vi "Coloring B-Scan Demo.vi"() -> ()   [LabVIEW 2012]
uses:
  LabVIEW/user.lib/SpectralRadar.llb/Color Enhancement Selection.ctl
  LabVIEW/user.lib/SpectralRadar.llb/Colorscheme Selection.ctl
  LabVIEW/user.lib/SpectralRadar.llb/Coloring Byteorder.ctl
  LabVIEW/user.lib/SpectralRadar.llb/Device Camera Preset Selection.ctl
  LabVIEW/user.lib/SpectralRadar.llb/Processing Parameter Int Selection.ctl
  LabVIEW/user.lib/SpectralRadar.llb/Probe Parameter Int Selection.ctl
  LabVIEW/user.lib/SpectralRadar.llb/Colored Data Export Format Selection.ctl
  LabVIEW/user.lib/SpectralRadar.llb/set Transposed Colored Scan Output.vi
  LabVIEW/user.lib/SpectralRadar.llb/set Scan Output.vi
  LabVIEW/user.lib/SpectralRadar.llb/Data.lvclass
  LabVIEW/user.lib/SpectralRadar.llb/OCT Device.lvclass
  LabVIEW/user.lib/SpectralRadar.llb/Probe.lvclass
  LabVIEW/user.lib/SpectralRadar.llb/Processing.lvclass
  LabVIEW/user.lib/SpectralRadar.llb/Raw Data.lvclass
  LabVIEW/user.lib/SpectralRadar.llb/Scan Pattern.lvclass
  LabVIEW/user.lib/SpectralRadar.llb/Coloring.lvclass
  LabVIEW/user.lib/SpectralRadar.llb/Colored Data.lvclass
  <vilib>/Analysis/NI_AALBase.lvlib
  <vilib>/Analysis/NI_AALPro.lvlib
  LabVIEW/user.lib/SpectralRadar.llb/LabVIEW Helper.lvlib
panel:
  in  "Save Button":bool
  in  "File Name":path
  in  "Display On/Off":bool
  in  "Range":dbl=1.0
  in  "Show Histogram":bool
  in  "Equalize":bool
  out "XY Graph 2":cluster{"X Values":dbl[], "Integral X":dbl[]}(graph)
  in  "Autoscale":bool
  out "XY Graph":T1(graph)
  in  "Color Table Selection":T2
  out "Averaged Frame Rate":dbl=6.134969234466553 format="%#_3g"
  out "Current Frame Rate":dbl=6.134969234466553 format="%#_3g"
  in  "Color Enhancement":T3
  in  "Boundries":cluster{sgl, sgl}(slide)={76.65738, 42.00557} scale=-20.0..120.0
  out "Image":T4(plugin-control)
  in  "stop":bool
  in  "AScans":i32=1024
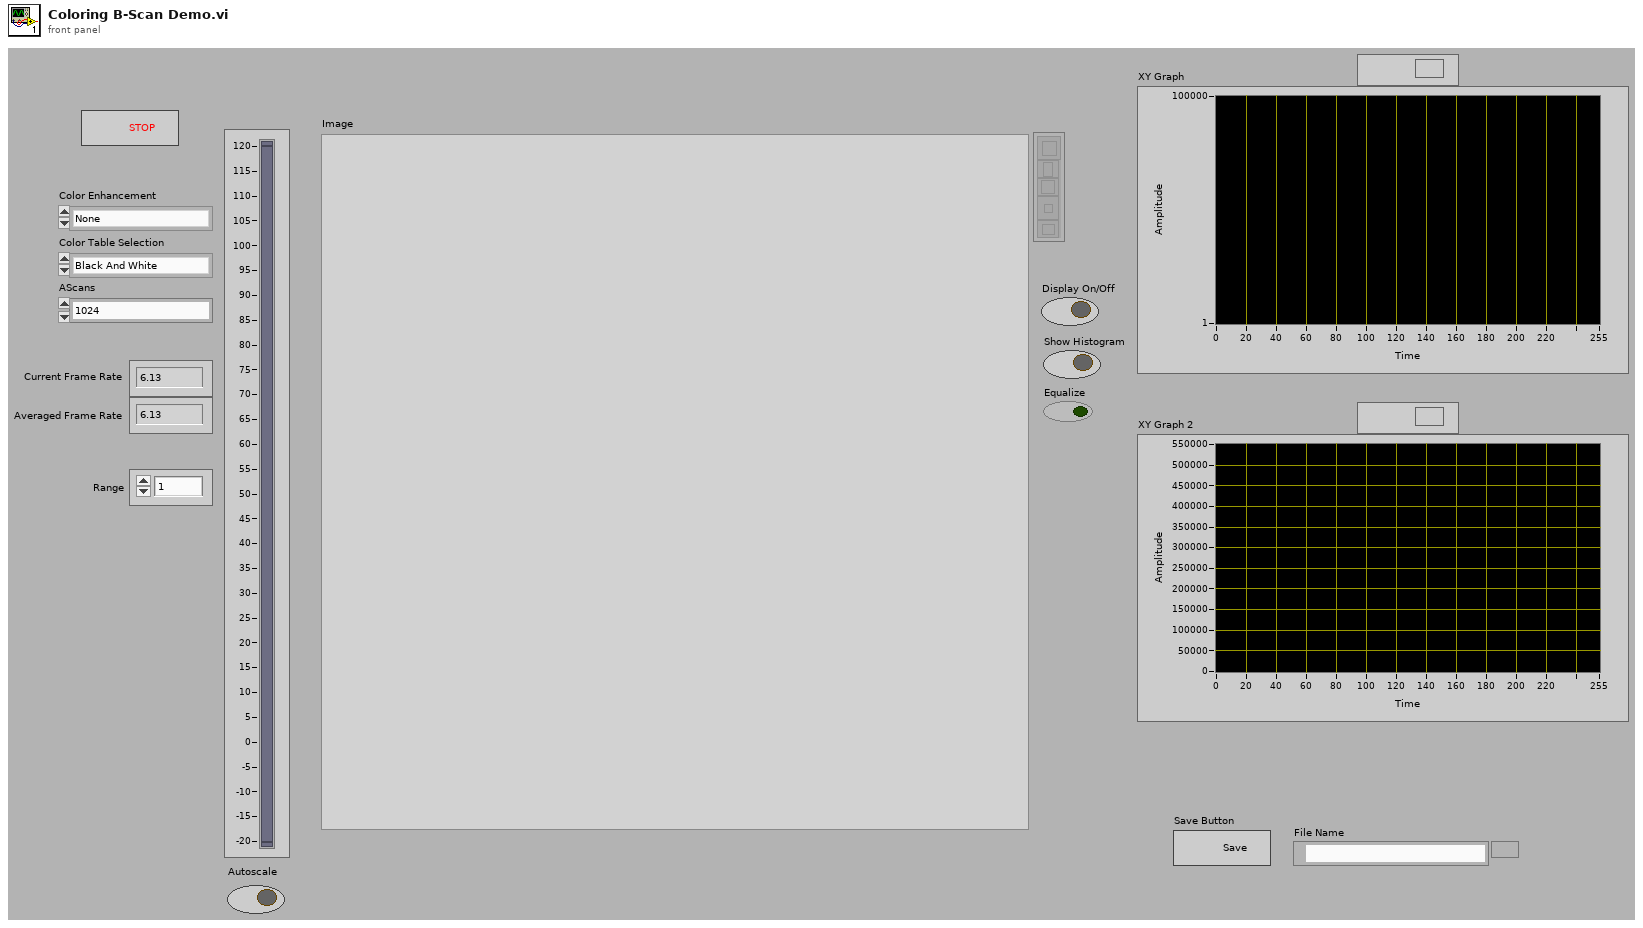
[diagram p1: front panel]
types:
  T1 = cluster{"X Values":dbl[], "Histogram: h(x)":i32[]}
  T2 = typedef "Coloring.lvclass/Colorscheme Selection.ctl" = enum16{"Black And White", "Inverted Black And White", "Color", "Black and Orange", "Black and Red", "Doppler Phase Coloring"}
  T3 = typedef "Coloring.lvclass/Color Enhancement Selection.ctl" = enum16{"None", "Sine", "Parable", "Cubic", "Square Root"}
  T4 = typedef "IMAQ Image.ctl" = refnum<image>
  T5 = typedef "Probe.lvclass/Probe Parameter Int Selection.ctl" = enum16{"Apodization Cycles", "Oversampling", "Oversampling Slow Axis", "Speckle Reduction"}
  T6 = typedef "Processing.lvclass/Processing Parameter Int Selection.ctl" = enum32{"Spectrum Averaging", "A-Scan Averaging", "B-Scan Averaging", "Zero Padding", "Number of Threads", "Fourier Averaging"}
  T7 = typedef "OCT Device.lvclass/Device Camera Preset Selection.ctl" = enum16{"Default", "Preset 1", "Preset 2", "Preset 3"}
  T8 = typedef "Coloring.lvclass/Coloring Byteorder.ctl" = enum16{"RGBA32", "BGRA32", "ARGB32", ""}
  T9 = typedef "Image Type" = u32
  T10 = enum16{"Asynchronous Continuous", "Asynchronous Finite", "Synchronous"}
  T11 = typedef "Colored Data.lvclass/Colored Data Export Format Selection.ctl" = enum16{"SRM (Spectral Radar Metafile)", "RAW", "BMP", "PNG", "JPG", "PDF", "TIFF"}
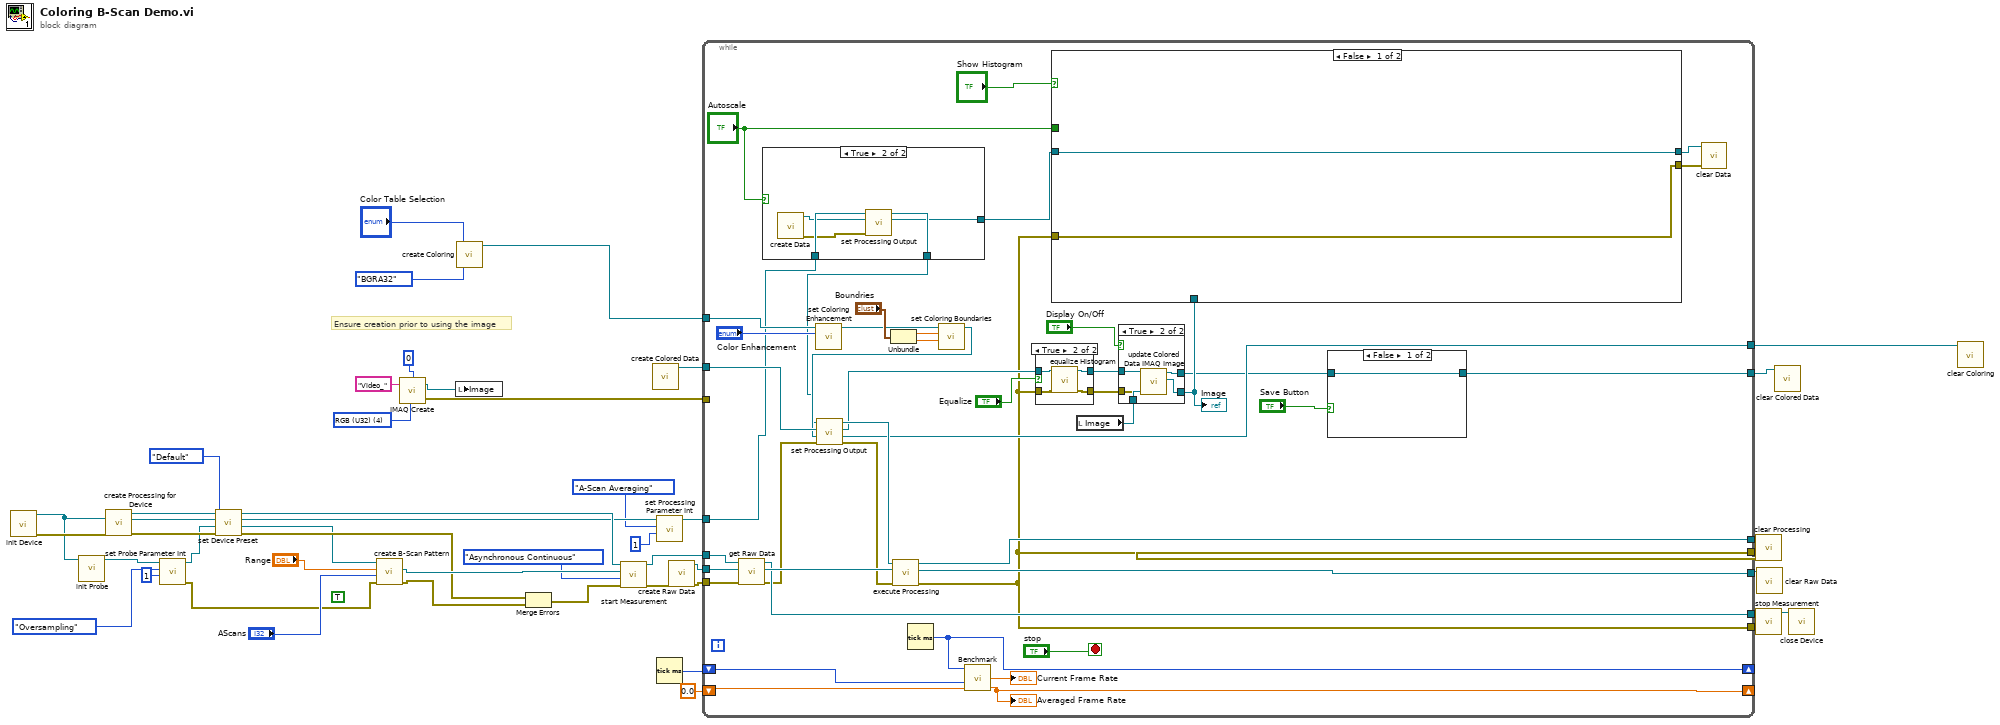
[diagram p0: block diagram]
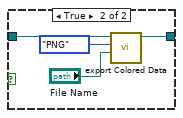
[diagram p2: hidden frame]
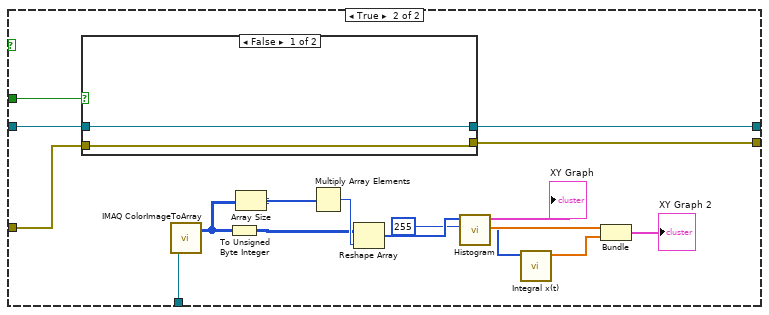
[diagram p4: hidden frame]
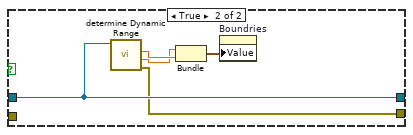
[diagram p5: hidden frame]
diagram:
  (unwired) TRUE
  w26 = T9 4 items=["Grayscale (U8)", "Grayscale (I16)", "Grayscale (SGL)", "Complex (CSG)", "RGB (U32)", "HSL (U32)", "RGB (U64)", "Grayscale (U16)"] ("Image Type")
  # "Ensure creation prior to using the image"
  n1 = call "init Device.vi"() -> ("error out"=w45:errorcluster, "OCTDevice"=w14:refnum<class "OCT Device.lvclass">)  [unwired: 6 in]
  n2 = call "init Probe.vi"("OCT Device"=w14) -> ("GalvoControl"=w6:refnum<class "Probe.lvclass">)  [unwired: 5 in, 1 out]
  n3 = call "create Processing for Device.vi"("error in (no error)"=w45, "OCTDevice"=w14) -> ("error out"=w39:errorcluster, "Processing"=w17:refnum<class "Processing.lvclass">, "OCTDevice"=w18:refnum<class "OCT Device.lvclass">)  [unwired: 3 in]
  n4 = call "set Probe Parameter Int.vi"("Value"=1, "Probe Parameter Int"=Probe_Parameter_Int_Selection."Oversampling", "GalvoControl"=w6) -> ("error out"=w4:errorcluster, "GalvoControl"=w5:refnum<class "Probe.lvclass">)  [unwired: 3 in]
  n5 = call "set Device Preset.vi"("Numeric"=Device_Camera_Preset_Selection."Default" ("Device Camera Preset Selection"), "Probe"=w5, "Processing"=w17, "OCTDevice"=w18) -> ("Probe 2"=w13:refnum<class "Probe.lvclass">, "Processing"=w11:refnum<class "Processing.lvclass">, "OCTDevice out"=w16:refnum<class "OCT Device.lvclass">)  [unwired: 2 in, 1 out]
  n6 = call "create B-Scan Pattern.vi"("error in (no error)"=w4, "AScans"="AScans", "Range"="Range", "Probe"=w13) -> ("error out"=w41:errorcluster, "Scan Pattern"=w43:refnum<class "Scan Pattern.lvclass">)  [unwired: 2 in, 1 out]
  n7 = call "IMAQ Create"("Border Size"=0, "Image Name"="Video_", "Image Type"=w26) -> ("New Image"=w24:T4, "error out"=w20:errorcluster)  [unwired: 2 in]
  n8 = local write "Image"(w24) -> ()
  n9 = call "create Coloring.vi"("Color Byte Order"=Coloring_Byteorder."BGRA32", "Color Table Selection"="Color Table Selection") -> ("Coloring"=w23:refnum<class "Coloring.lvclass">)  [unwired: 4 in, 1 out]
  n10 = Merge Errors(w39, w41) -> (w40:errorcluster)
  n11 = call "start Measurement.vi"("error in (no error)"=w40, "Acquisition Type"=T10."Asynchronous Continuous", "Scan Pattern"=w43, "OCTDevice"=w16) -> ("error out"=w37:errorcluster, "OCTDevice"=w30:refnum<class "OCT Device.lvclass">)  [unwired: 1 in, 1 out]
  n12 = call "create Colored Data.vi"() -> ("Colored Data"=w28:refnum<class "Colored Data.lvclass">)  [unwired: 6 in, 1 out]
  n13 = call "set Processing Parameter Int.vi"("Value"=1, "Processing Paramter Int Selection"=Processing_Parameter_Int_Selection."A-Scan Averaging", "Processing in"=w11) -> ("Processing out"=w10:refnum<class "Processing.lvclass">)  [unwired: 3 in, 1 out]
  n14 = Tick Count (ms)() -> (millisecond timer value=w22:u32)
  n15 = call "create Raw Data.vi"("error in (no error)"=w37) -> ("error out"=w36:errorcluster, "Raw Data"=w38:refnum<class "Raw Data.lvclass">)  [unwired: 5 in]
  n16 = while {
    tunnel: w38 -> [w87]
    tunnel: w30 -> [w88]
    tunnel: w36 -> [w86]
    tunnel: w10 -> [w64]
    tunnel: [w83] -> w35
    tunnel: [w82] -> w34
    tunnel: [w81] -> w32
    tunnel: [w57] -> w33
    tunnel: [w57] -> _
    tunnel: w28 -> [w67]
    tunnel: w23 -> [w71]
    shift-right: [w68] -> _
    shift-left: w22 -> [w70]
    tunnel: [w65] -> w21
    tunnel: w20 -> [_]
    shift-right: [w54] -> _
    shift-left: sgl 0.0 ("AverageFrameRate") -> [w53]
    tunnel: [w49] -> w7
    stop <- "stop" stop-if-true
    n17 = call "get Raw Data.vi"("error in (no error)"=w86, "RawData in"=w87, "OCTDevice in"=w88) -> ("error out"=w80:errorcluster, "RawData out"=w84:refnum<class "Raw Data.lvclass">, "OCTDevice out"=w81:refnum<class "OCT Device.lvclass">)  [unwired: 2 in]
    n18 = case shown="True" "Autoscale" {
      tunnel: w64 -> [w133 w138]
      tunnel: [w133 w137] -> w63
      tunnel: [_ w136] -> w62
      frame False {
      }
      frame True {
        n19 = call "create Data.vi"() -> ("error out"=w134:errorcluster, "Data"=w135:refnum<class "Data.lvclass">)  [unwired: 6 in]
        n20 = call-poly "set Processing Output.vi"("error in (no error)"=w134, "Data"=w135, "Processing"=w138) -> ("Data"=w136:refnum<class "Data.lvclass">, "Processing"=w137:refnum<class "Processing.lvclass">)  [unwired: 2 in, 1 out]
      }
    }
    n21 = call "set Coloring Enhancement.vi"("Color Enhancement"="Color Enhancement", "Coloring in"=w71) -> ("Coloring out"=w72:refnum<class "Coloring.lvclass">)  [unwired: 4 in, 1 out]
    n22 = Unbundle("Boundries") -> (w75:sgl, w74:sgl)
    n23 = Tick Count (ms)() -> (millisecond timer value=w68:u32)
    n24 = call "set Coloring Boundaries.vi"("Danymic Range High [dB]"=w74, "Dynamic Range Low [dB]"=w75, "Coloring in"=w72) -> ("Coloring out"=w66:refnum<class "Coloring.lvclass">)  [unwired: 3 in, 1 out]
    n25 = call-poly "set Processing Output.vi"("error in (no error)"=w80, "Coloring"=w66, "Colored Data"=w67, "Processing"=w63) -> ("error out"=w78:errorcluster, "Coloring"=w65:refnum<class "Coloring.lvclass">, "Colored Data"=w60:refnum<class "Colored Data.lvclass">, "Processing"=w85:refnum<class "Processing.lvclass">)
    n26 = call "execute Processing.vi"("error in (no error)"=w78, "Raw Data"=w84, "Processing"=w85) -> ("error out"=w57:errorcluster, "Raw Data"=w83:refnum<class "Raw Data.lvclass">, "Processing"=w82:refnum<class "Processing.lvclass">)  [unwired: 2 in]
    n27 = call "Benchmark.vi"("Last Frame Rate"=w53, "TimeStart"=w70, "TimeFinish"=w68) -> ("AverageFrameRate"=w54:sgl, "FrameRate"=→"Current Frame Rate":sgl)  [unwired: 1 in, 1 out]
    "Averaged Frame Rate" <- w54
    n28 = case shown="True" "Equalize" {
      tunnel: w60 -> [w127 w132]
      tunnel: [w127 w131] -> w59
      tunnel: w57 -> [w128 w130]
      tunnel: [w128 w129] -> w56
      frame False {
      }
      frame True {
        n29 = call "equalize Histogram.vi"("error in (no error)"=w130, "Colored Data in"=w132) -> ("error out"=w129:errorcluster, "Colored Data out"=w131:refnum<class "Colored Data.lvclass">)  [unwired: 4 in]
      }
    }
    n30 = local read "Image"() -> (w77:T4)
    n31 = case shown="True" "Display On/Off" {
      tunnel: w77 -> [w95 w100]
      tunnel: w59 -> [w94 w99]
      tunnel: w56 -> [_ w98]
      tunnel: [w94 w97] -> w50
      tunnel: [w95 w96] -> w51
      frame False {
      }
      frame True {
        n32 = call "update Colored Data IMAQ Image.vi"("error in (no error)"=w98, "Image in"=w100, "Colored Data"=w99) -> ("Image out"=w96:T4, "Colored Data"=w97:refnum<class "Colored Data.lvclass">)  [unwired: 2 in, 1 out]
      }
    }
    "Image" <- w51
    n33 = case shown="False" "Show Histogram" {
      tunnel: w51 -> [_ w119]
      tunnel: w62 -> [w102 w112]
      tunnel: "Autoscale" -> [_ w111]
      tunnel: w57 -> [w101 w105]
      tunnel: [w102 w104] -> w47
      tunnel: [w101 w103] -> w46
      frame False {
      }
      frame True {
        n34 = case shown="False" w111 {
          tunnel: w105 -> [w121 _]
          tunnel: w112 -> [w120 w123]
          tunnel: [w120 w123] -> w104
          tunnel: [w121 w122] -> w103
          frame False {
          }
          frame True {
            n35 = call "determine Dynamic Range.vi"("Data in"=w123) -> ("error out"=w122:errorcluster, "High"=w124:sgl, "Low"=w125:sgl)  [unwired: 3 in, 1 out]
            n36 = Bundle("High"=w124, "Low"=w125) -> (w126:cluster{"High":sgl, "Low":sgl})  [unwired: 1 in]
            n37 = property on="Boundries" class="Slide (strict)"("Value"=w126) -> ()  [unwired: 2 in, 2 out]
          }
        }
        n38 = call "IMAQ ColorImageToArray"("Image"=w119) -> ("Image Pixels (U32)"=w114:u32[][])  [unwired: 3 in, 2 out]
        n39 = To Unsigned Byte Integer(number=w114) -> (unsigned 8bit integer=w113:u8[][])
        n40 = Array Size(array=w114) -> (size(s)=w116:i32[])
        n41 = Multiply Array Elements(1:w116) -> (0:w115:i32)
        n42 = Reshape Array(w113, w115) -> (w118:u8[])
        n43 = call <vilib>:"Histogram.vi"("intervals"=255, "X"=w118) -> ("X Values"=w109:dbl[], "Histogram: h(x)"=w108:i32[], "Histogram Graph"=→"XY Graph":T1)  [unwired: 6 in, 1 out]
        n44 = call <vilib>:"Integral x(t).vi"("X"=w108) -> ("Integral X"=w107:dbl[])  [unwired: 9 in, 1 out]
        n45 = Bundle("X Values"=w109, "Integral X"=w107) -> (→"XY Graph 2":cluster{"X Values":dbl[], "Integral X":dbl[]})  [unwired: 1 in]
      }
    }
    n46 = case shown="False" "Save Button" {
      tunnel: w50 -> [w89 w93]
      tunnel: [w89 w92] -> w49
      frame False {
      }
      frame True {
        n47 = call "export Colored Data.vi"("File Name"="File Name", "Colored Data Export Format Selection"=Colored_Data_Export_Format_Selection."PNG", "Colored Data in"=w93) -> ("Colored Data out"=w92:refnum<class "Colored Data.lvclass">)  [unwired: 3 in, 1 out]
      }
    }
    n48 = call "clear Data.vi"("error in (no error)"=w46, "Data"=w47) -> ()  [unwired: 5 in, 1 out]
  }
  n49 = call "clear Processing.vi"("error in (no error)"=w33, "Processing"=w34) -> ()  [unwired: 5 in, 1 out]
  n50 = call "stop Measurement.vi"("OCTDevice"=w32) -> ("OCTDevice"=w31:refnum<class "OCT Device.lvclass">)  [unwired: 5 in, 1 out]
  n51 = call "clear Raw Data.vi"("Raw Data"=w35) -> ()  [unwired: 6 in, 1 out]
  n52 = call "clear Colored Data.vi"("Colored Data"=w7) -> ()  [unwired: 6 in, 1 out]
  n53 = call "close Device.vi"("OCTDevice"=w31) -> ()  [unwired: 6 in, 1 out]
  n54 = call "clear Coloring.vi"("Coloring"=w21) -> ()  [unwired: 6 in, 1 out]
